vi "HW_GEN_Handle Sync Data.vi"(8 "error in":errorcluster, 11 "Data in":cluster{"Values":dbl[], "Timestamps":dbl[]}[](array[cluster])) -> (0 "error out":errorcluster, 2 "Samples per CH":i32, 3 "Data out":cluster{"Values":dbl[], "Timestamps":dbl[]}[](array[cluster]))   [LabVIEW 2016]
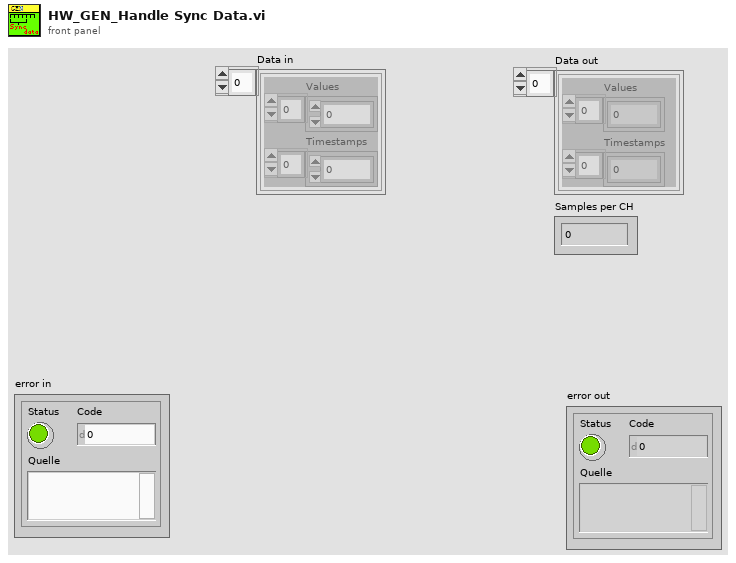
[diagram p1: front panel]
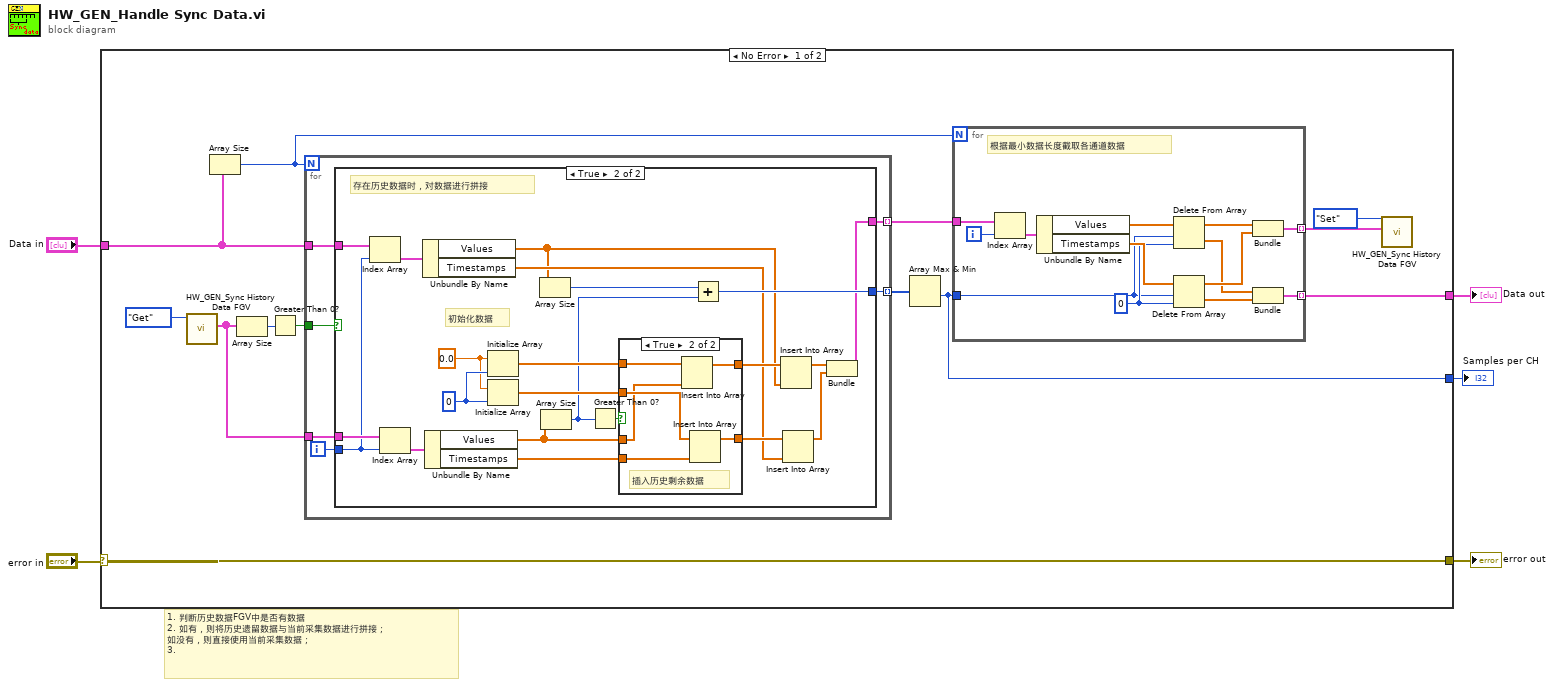
[diagram p0: block diagram]
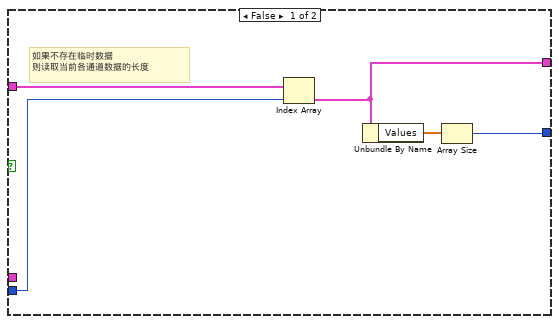
[diagram p2: hidden frame]
diagram:
  # "1. 判断历史数据FGV中是否有数据\n2. 如有，则将历史遗留数据与当前采集数据进行拼接；\n如没有，则直接使用当前采集数据；\n3."
  n1 = case shown="No Error" "error in" {
    selector: "error in" -> [w18 w74]
    tunnel: [w18 w74] -> w4
    tunnel: "Data in" -> [w15 w73]
    tunnel: [w7 w73] -> w2
    tunnel: [w6 _] -> w1
    frame No Error {
      n2 = call "HW_GEN_Sync History Data FGV.vi"("Mode"=enum16{"Get", "Set", "Init"}."Get") -> ("Data Blocks out"=w9:cluster{"Values":dbl[], "Timestamps":dbl[]}[])  [unwired: 10 in]
      n3 = Array Size(array=w15) -> (size(s)=w14:i32)
      n4 = Array Size(array=w9) -> (size(s)=w17:i32)
      n5 = Greater Than 0?(x=w17) -> (x > 0?=w16:bool)
      n6 = for {
        N: w14 -> [_]
        tunnel: w15 -> [w36]
        tunnel: w16 -> [w37]
        tunnel: w9 -> [w35]
        tunnel: [w34] -> w13 mode=indexing
        tunnel: [w32] -> w8 mode=indexing
        i -> [w33]
        n7 = case shown="True" w37 {
          tunnel: w36 -> [w42 w64]
          tunnel: w33 -> [w41 w61]
          tunnel: [w40 w43] -> w34
          tunnel: w35 -> [_ w62]
          tunnel: [w38 w56] -> w32
          frame False {
            # "如果不存在临时数据\n则读取当前各通道数据的长度"
            n8 = Index Array(array=w42, index=w41) -> (element=w40:cluster{"Values":dbl[], "Timestamps":dbl[]})
            n9 = Unbundle By Name(w40) -> ("Values"=w39:dbl[])
            n10 = Array Size(array=w39) -> (size(s)=w38:i32)
          }
          frame True {
            w54 = 0.0
            w55 = 0 ("Dimension")
            # "初始化数据"
            # "存在历史数据时，对数据进行拼接"
            n11 = Index Array(array=w64, index=w61) -> (element=w63:cluster{"Values":dbl[], "Timestamps":dbl[]})
            n12 = Index Array(array=w62, index=w61) -> (element=w60:cluster{"Values":dbl[], "Timestamps":dbl[]})
            n13 = Unbundle By Name(w63) -> ("Values"=w46:dbl[], "Timestamps"=w50:dbl[])
            n14 = Unbundle By Name(w60) -> ("Values"=w47:dbl[], "Timestamps"=w48:dbl[])
            n15 = Initialize Array(w54, w55) -> (w53:dbl[])
            n16 = Initialize Array(w54, w55) -> (w58:dbl[])
            n17 = Array Size(array=w46) -> (size(s)=w51:i32)
            n18 = Array Size(array=w47) -> (size(s)=w49:i32)
            n19 = Greater Than 0?(x=w49) -> (x > 0?=w59:bool)
            n20 = case shown="True" w59 {
              tunnel: w58 -> [w65 w70]
              tunnel: [w66 w71] -> w57
              tunnel: w53 -> [w66 w72]
              tunnel: w47 -> [_ w68]
              tunnel: w48 -> [_ w69]
              tunnel: [w65 w67] -> w52
              frame False {
                # "没有历史数据"
              }
              frame True {
                # "插入历史剩余数据"
                n21 = Insert Into Array(array=w72, new element=w68) -> (w71:dbl[])  [unwired: 1 in]
                n22 = Insert Into Array(array=w70, new element=w69) -> (w67:dbl[])  [unwired: 1 in]
              }
            }
            n23 = Add(x=w51, y=w49) -> (x+y=w56:i32)
            n24 = Insert Into Array(array=w57, new element=w46) -> (w45:dbl[])  [unwired: 1 in]
            n25 = Insert Into Array(array=w52, new element=w50) -> (w44:dbl[])  [unwired: 1 in]
            n26 = Bundle(w45, w44) -> (w43:cluster{dbl[], dbl[]})  [unwired: 1 in]
          }
        }
      }
      n27 = Array Max & Min(array=w8) -> (min value=w6:i32)  [unwired: 3 out]
      n28 = for {
        N: w14 -> [_]
        tunnel: w13 -> [w30]
        tunnel: [w28] -> w12 mode=indexing
        tunnel: w6 -> [w22]
        tunnel: [w19] -> w7 mode=indexing
        i -> [w27]
        w24 = 0 ("Index")
        # "根据最小数据长度截取各通道数据"
        n29 = Index Array(array=w30, index=w27) -> (element=w31:cluster{"Values":dbl[], "Timestamps":dbl[]})
        n30 = Unbundle By Name(w31) -> ("Values"=w26:dbl[], "Timestamps"=w25:dbl[])
        n31 = Delete From Array(array=w26, length=w22, index=w24) -> (deleted portion=w21:dbl[], array with subset deleted=w29:dbl[])
        n32 = Delete From Array(array=w25, length=w22, index=w24) -> (deleted portion=w20:dbl[], array with subset deleted=w23:dbl[])
        n33 = Bundle("Values"=w29, "Timestamps"=w23) -> (w28:cluster{"Values":dbl[], "Timestamps":dbl[]})  [unwired: 1 in]
        n34 = Bundle("Values"=w21, "Timestamps"=w20) -> (w19:cluster{"Values":dbl[], "Timestamps":dbl[]})  [unwired: 1 in]
      }
      n35 = call "HW_GEN_Sync History Data FGV.vi"("Data Blocks in"=w12, "Mode"=enum16{"Get", "Set", "Init"}."Set") -> ()  [unwired: 9 in, 1 out]
    }
    frame Error {
    }
  }
  "error out" <- w4
  "Data out" <- w2
  "Samples per CH" <- w1
